vi "64 Bit to 128 Bit Bundle (SubVI).vi"(9 "Data Valid?":bool, 11 "Data In":u64) -> (0 "Output Valid?":bool, 3 "Data Out":T1)   [LabVIEW 2015]
uses:
  Controls (FPGA)/Pixel Bundle (x16).ctl
  Controls (FPGA)/Pack Cam Data.ctl
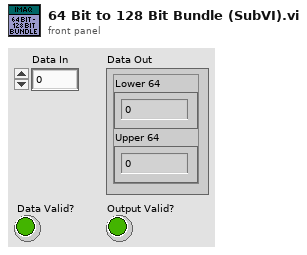
[diagram p1: front panel]
types:
  T1 = typedef "Pixel Bundle (x16).ctl" = cluster{"Lower 64":u64, "Upper 64":u64}
  T2 = typedef "Pack Cam Data.ctl" = enum16{"Read Lower 64", "Read Upper 64"}
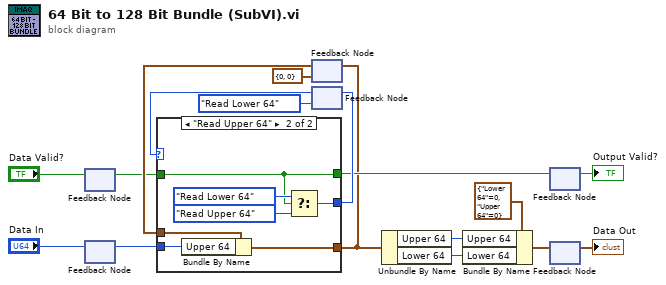
[diagram p0: block diagram]
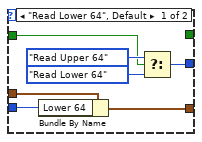
[diagram p2: hidden frame]
diagram:
  n1 = feedback-in #1("Data Valid?") -> ()
  n2 = feedback #1() -> (w9:bool)  [unwired: 1 in]
  n3 = feedback-in #2("Data In") -> ()
  n4 = feedback #2() -> (w8:u64)  [unwired: 1 in]
  n5 = feedback #3(cluster{"Upper 64":u64, "Lower 64":u64} {"Upper 64"=0, "Lower 64"=0} ("Element")) -> (w11:cluster{"Upper 64":u64, "Lower 64":u64})
  n6 = feedback #4(Pack_Cam_Data."Read Lower 64") -> (w13:T2)
  n7 = case shown="\"Read Upper 64\"" w13 {
    tunnel: [w22 w29] -> w14
    tunnel: w8 -> [w20 w28]
    tunnel: w9 -> [w21 w25]
    tunnel: [w19 w27] -> w5
    tunnel: w11 -> [w18 w26]
    tunnel: [_ w25] -> w10
    frame "Read Lower 64", Default {
      n8 = Bundle By Name(cluster=w18, "Lower 64"=w20) -> (w19:cluster{"Upper 64":u64, "Lower 64":u64})
      n9 = Select(t=Pack_Cam_Data."Read Upper 64", s=w21, f=Pack_Cam_Data."Read Lower 64") -> (s? t:f=w22:T2)
    }
    frame "Read Upper 64" {
      n10 = Bundle By Name(cluster=w26, "Upper 64"=w28) -> (w27:cluster{"Upper 64":u64, "Lower 64":u64})
      n11 = Select(t=Pack_Cam_Data."Read Lower 64", s=w25, f=Pack_Cam_Data."Read Upper 64") -> (s? t:f=w29:T2)
    }
  }
  n12 = feedback-in #3(w5) -> ()
  n13 = feedback-in #4(w14) -> ()
  n14 = Unbundle By Name(w5) -> ("Upper 64"=w4:u64, "Lower 64"=w1:u64)
  n15 = Bundle By Name(cluster=T1 {"Lower 64"=0, "Upper 64"=0} ("Pixel Bundle (x16)"), "Upper 64"=w4, "Lower 64"=w1) -> (w3:T1)
  n16 = feedback-in #5(w10) -> ()
  n17 = feedback #5() -> (→"Output Valid?":bool)  [unwired: 1 in]
  n18 = feedback-in #6(w3) -> ()
  n19 = feedback #6() -> (→"Data Out":T1)  [unwired: 1 in]
